vi "Configure Current Range.vi"(0 "VISA resource name":refnum<visa-resource-name>, 1 "Autorange (T: Enable)":bool=TRUE, 5 "Auto Range Max (20mA)":u16(ring) items=["20mA", "2mA", "200uA", "20uA", "2uA", "200nA", "20nA", "2nA"], 7 "Auto Range Min (2nA)":u16(ring)=7 items=["20mA", "2mA", "200uA", "20uA", "2uA", "200nA", "20nA", "2nA"], 9 "Upper Measurement Range (200uA)":u16(ring)=2 items=["20mA", "2mA", "200uA", "20uA", "2uA", "200nA", "20nA", "2nA"], 11 "error in (no error)":errorcluster) -> (4 "VISA resource name out":refnum<visa-resource-name>, 15 "error out":errorcluster)   [LabVIEW 2020, in "Keithley 648X Series.lvlib"]
doc: "Configures the current autorange or the upper current measurement range."
uses:
  <instrlib>/Keithley 648X Series/Keithley 648X Series.lvlib
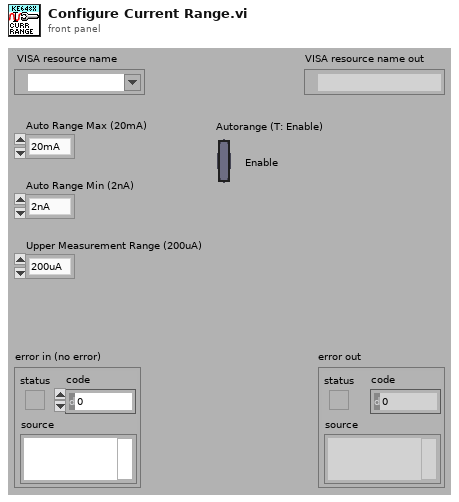
[diagram p1: front panel]
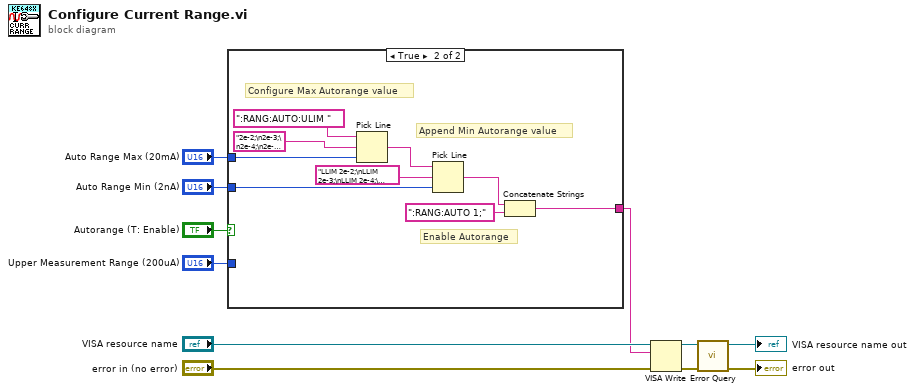
[diagram p0: block diagram]
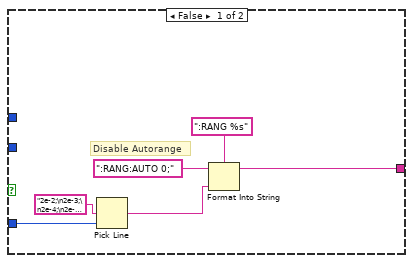
[diagram p2: hidden frame]
diagram:
  n1 = case shown="True" "Autorange (T: Enable)" {
    tunnel: "Auto Range Max (20mA)" -> [_ w24]
    tunnel: "Auto Range Min (2nA)" -> [_ w21]
    tunnel: [w12 w18] -> w2
    tunnel: "Upper Measurement Range (200uA)" -> [w15 _]
    frame False {
      # "Disable Autorange"
      n2 = Pick Line(multi-line string="2e-2;\n2e-3;\n2e-4;\n2e-5;\n2e-6;\n2e-7;\n2e-8;\n2e-9;", line index=w15) -> (output string=w14:string)  [unwired: 1 in]
      n3 = Format Into String(format string=":RANG %s", initial string=":RANG:AUTO 0;", w14) -> (resulting string=w12:string)  [unwired: 1 in, 1 out]
    }
    frame True {
      # "Enable Autorange"
      # "Append Min Autorange value"
      # "Configure Max Autorange value"
      n4 = Pick Line(string ("")=":RANG:AUTO:ULIM ", multi-line string="2e-2;\n2e-3;\n2e-4;\n2e-5;\n2e-6;\n2e-7;\n2e-8;\n2e-9;", line index=w24) -> (output string=w23:string)
      n5 = Pick Line(string ("")=w23, multi-line string="LLIM 2e-2;\nLLIM 2e-3;\nLLIM 2e-4;\nLLIM 2e-5;\nLLIM 2e-6;\nLLIM 2e-7;\nLLIM 2e-8;\nLLIM 2e-9;", line index=w21) -> (output string=w20:string)
      n6 = Concatenate Strings(w20, ":RANG:AUTO 1;" ("string")) -> (w18:string)
    }
  }
  n7 = VISA Write(VISA resource name="VISA resource name", write buffer=w2, error in (no error)="error in (no error)") -> (VISA resource name out=w7:refnum<visa-resource-name>, error out=w6:errorcluster)  [unwired: 1 out]
  n8 = call <instrlib>:"Error Query.vi"("error in (no error)"=w6, "VISA resource name"=w7) -> ("error out"=→"error out":errorcluster, "VISA resource name out"=→"VISA resource name out":refnum<visa-resource-name>)  [unwired: 6 in, 2 out]
